vi "proc.util.validateParamExist.vi"(7 "format string":string="Missing required step parameter (%s)", 8 "error in":errorcluster, 9 "isRequired":bool, 10 "Param Label":string, 11 "isFound":bool) -> (0 "error out":errorcluster)   [LabVIEW 2024]
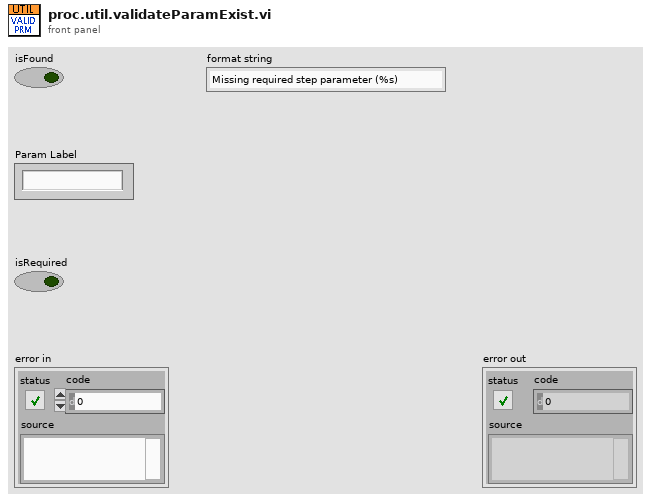
[diagram p1: front panel]
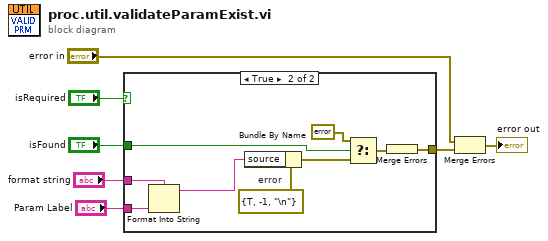
[diagram p0: block diagram]
diagram:
  n1 = case shown="True" "isRequired" {
    tunnel: "isFound" -> [_ w16]
    tunnel: [_ w8] -> w4
    tunnel: "Param Label" -> [_ w9]
    tunnel: "format string" -> [_ w10]
    frame False {
    }
    frame True {
      w13 = errorcluster {"status"=TRUE, "code"=-1, "source"="\n"}  # error
      n2 = Format Into String(format string=w10, w9) -> (resulting string=w14:string)  [unwired: 2 in, 1 out]
      n3 = Bundle By Name(cluster=w13, "source"=w14) -> (w12:errorcluster)
      n4 = Select(t=errorcluster {"status"=FALSE, "code"=0, "source"=""}, s=w16, f=w12) -> (s? t:f=w15:errorcluster)
      n5 = Merge Errors(w15) -> (w8:errorcluster)
    }
  }
  n6 = Merge Errors("error in", w4) -> (→"error out":errorcluster)
